vi "Cancel Calling VI Wnd Topmost.vi"(8 "Error In":errorcluster) -> (0 "Error Out":errorcluster)   [LabVIEW 2015, in "Win32 Util.lvlib"]
doc: "Sets the Caller VIs front panel NoTopmost (above all non-topmost windows), thereby cancelling the TopMost setting.\n\nCopyright © 2010 Blue Ridge Test, Inc.\nwww.BlueRidgeTest.com"
uses:
  LabSDL2/Source/Libraries/Win32 Util/Win32 Util.lvlib
  USER32.DLL
panel:
  # "NP 2017-07-14\nTaken from\nhttps://lavag.org/topic/12751-how-do-you-make-your-application-window-frontmost/?do=findComment&comment=113072\n\nNot sure on copyright. Suspct this is public domain."
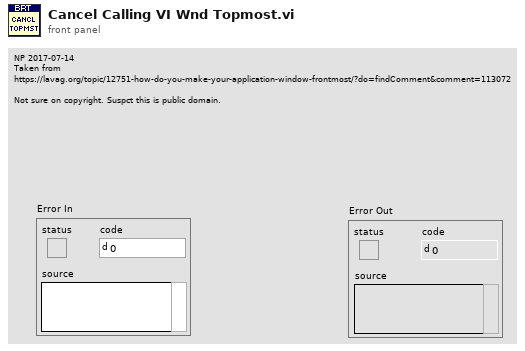
[diagram p1: front panel]
types:
  T1 = enum32{"Invalid", "Standard", "Closed", "Hidden", "Minimized", "Maximized"}
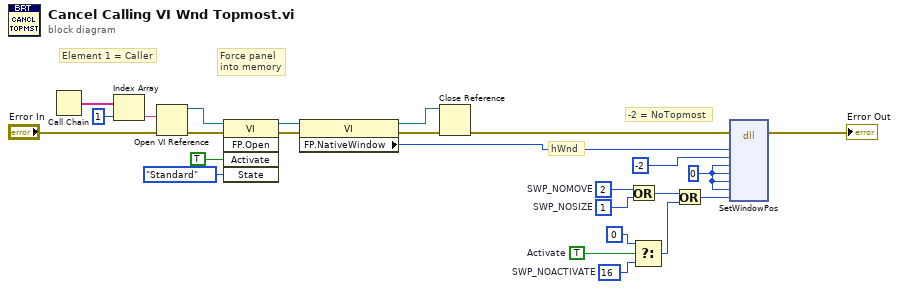
[diagram p0: block diagram]
diagram:
  w9 = TRUE  # Activate
  w10 = u32 2  # SWP_NOMOVE
  w11 = u32 1  # SWP_NOSIZE
  w12 = u32 16  # SWP_NOACTIVATE
  w8 = 0
  # "-2 = NoTopmost"
  # "hWnd"
  # "Force panel\ninto memory"
  # "Element 1 = Caller"
  n1 = Call Chain() -> (call chain=w22:string[])
  n2 = Index Array(array=w22, index=1) -> (element=w21:string)
  n3 = Open VI Reference(vi path=w21, error in (no error)="Error In") -> (vi reference=w18:refnum<vi>, error out=w19:errorcluster)  [unwired: 4 in]
  n4 = invoke class="VI" method="FP.Open"(reference=w18, error in=w19, "Activate"=TRUE ("Activate?"), "State"=T1."Standard") -> (reference out=w6:refnum<vi>, error out=w3:errorcluster)  [unwired: 1 in, 3 out]
  n5 = property class="VI"(reference=w6, error in=w3) -> (reference out=w2:refnum<vi>, error out=w1:errorcluster, "FP.NativeWindow"=w4:u64)
  n6 = Close Reference(reference=w2, error in (no error)=w1) -> (error out=w5:errorcluster)
  n7 = Or(x=w10, y=w11) -> (x .or. y?=w15:u32)
  n8 = Select(t=u32 0, s=w9, f=w12) -> (s? t:f=w14:u32)
  n9 = Or(x=w15, y=w14) -> (x .or. y?=w16:u32)
  n10 = dll-call lib="USER32.DLL" fn="SetWindowPos"(error in=w5, "hWnd"=w4, "hWndInsertAfter"=-2, "left"=w8, "top"=w8, "width"=w8, "height"=w8, "fuFlags"=w16) -> (error out=→"Error Out":errorcluster)  [unwired: 8 in, 3 out]
